vi "MacroEngine.vi"(11 "File Path":path=path "c:/RobotMacros.cfg") -> ()   [LabVIEW 2017]
uses:
  CtrlRefs/JoyStick1ALB.ctl
  CtrlRefs/JoyStick1ALV(Analog).ctl
  CtrlRefs/JoyStick2ALB.ctl
  CtrlRefs/JoyStick2ALB(Analog).ctl
  CtrlRefs/MacrosALB.ctl
  <vilib>/Rock Robotics/Network Tables/NT Write String Array.vi
  <vilib>/Rock Robotics/Network Tables/NT Write Boolean.vi
panel:
  out "MacroNames":string[](array[string])
  in  "DeleteMacroIndex":i32
  in  "DeleteMacro":bool
  in  "MacroRecStop":bool
  out "MacroRecording":bool
  out "MacroClock":dbl
  in  "MacroRecStart":bool
  in  "MacroName":string
  out "x*y":dbl
  out "Boolean":bool
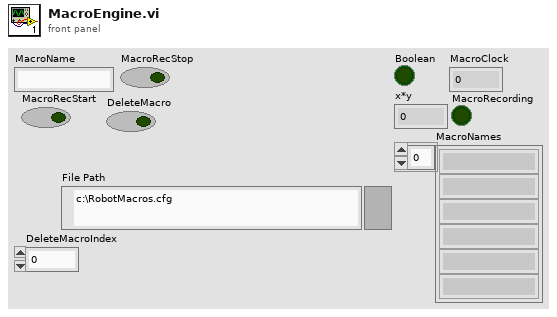
[diagram p1: front panel]
types:
  T1 = typedef "JoyStick1ALB.ctl" = cluster{"J1-B0":bool, "J1-B1":bool, "J1-B2":bool, "J1-B3":bool, "J1-B4":bool, "J1-B5":bool, "J1-B6":bool, "J1-B7":bool, "J1-B8-":bool, "J1-B9":bool, "J1-B10":bool, "J1-B11":bool}
  T2 = typedef "JoyStick1ALV(Analog).ctl" = cluster{"Axis 0":dbl, "Axis 1":dbl, "Axis 2":dbl, "Slider":dbl}
  T3 = typedef "JoyStick2ALB.ctl" = cluster{"J2-B0":bool, "J2-B1":bool, "J2-B2":bool, "J2-B3":bool, "J2-B4":bool, "J2-B5":bool, "J2-B6":bool, "J2-B7":bool, "J2-B8":bool, "J2-B9":bool, "J2-B10":bool, "J2-B11":bool}
  T4 = typedef "JoyStick2ALB(Analog).ctl" = cluster{"Axis 0":dbl, "Axis 1":dbl, "Axis 2":dbl, "Switch":dbl}
  T5 = cluster{"Buttons 1":T1, "Axes 1":T2, "Buttons 2":T3, "Axes 2":T4, "Delay":u32}
  T6 = cluster{"Buttons 1":T1, "Axes 1":T2, "Buttons 2":T3, "Axes 2":T4, "Delay":u32}[]
  T7 = typedef "MacrosALB.ctl" = cluster{"MacroName":string, "Sequence":cluster{"Buttons 1":T1, "Axes 1":T2, "Buttons 2":T3, "Axes 2":T4, "Delay":u32}[], "TotalTime":u32}
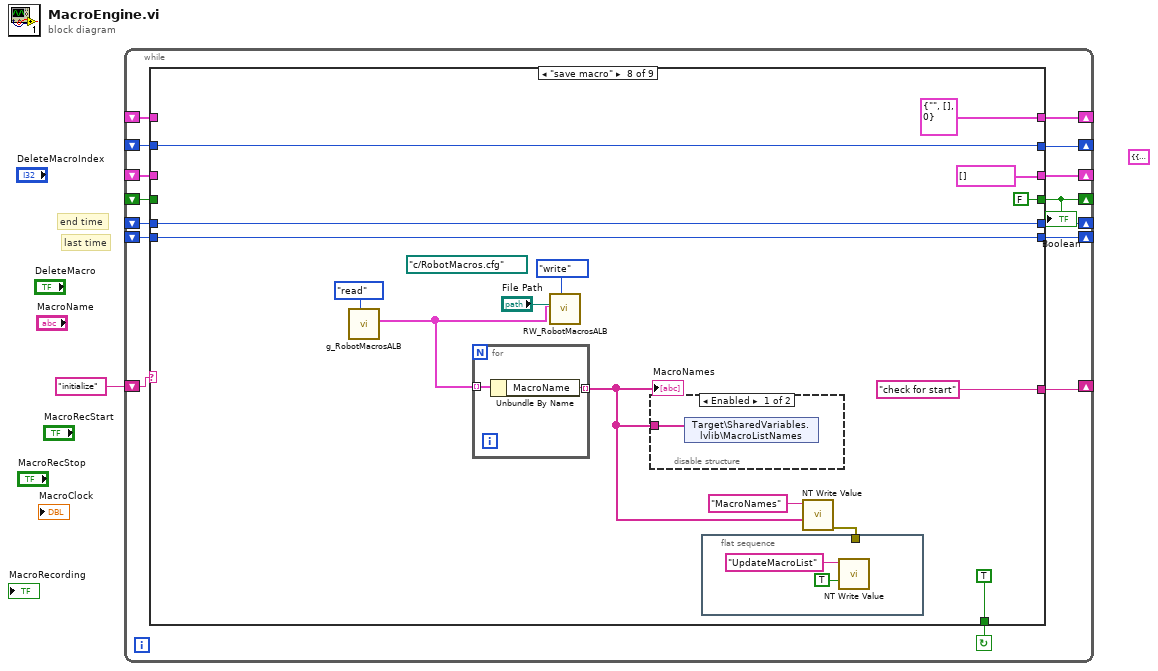
[diagram p0: block diagram]
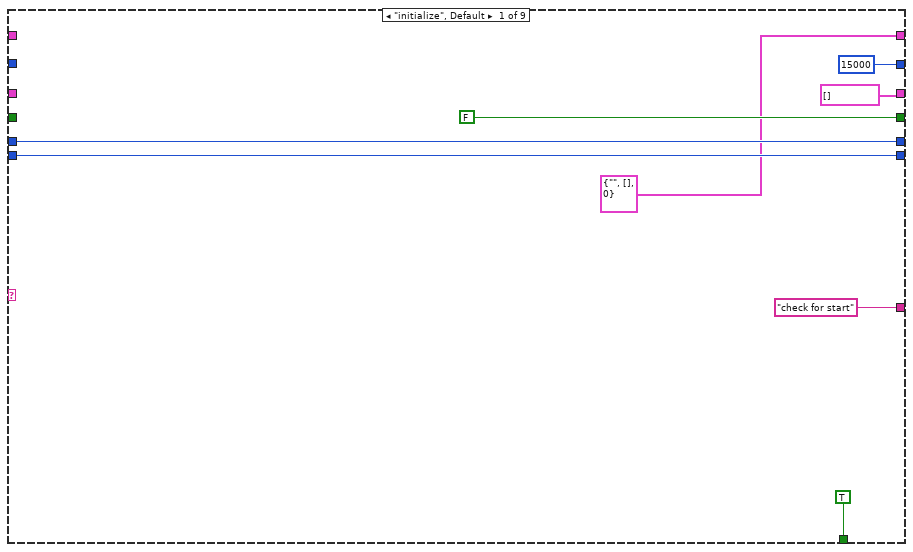
[diagram p2: hidden frame]
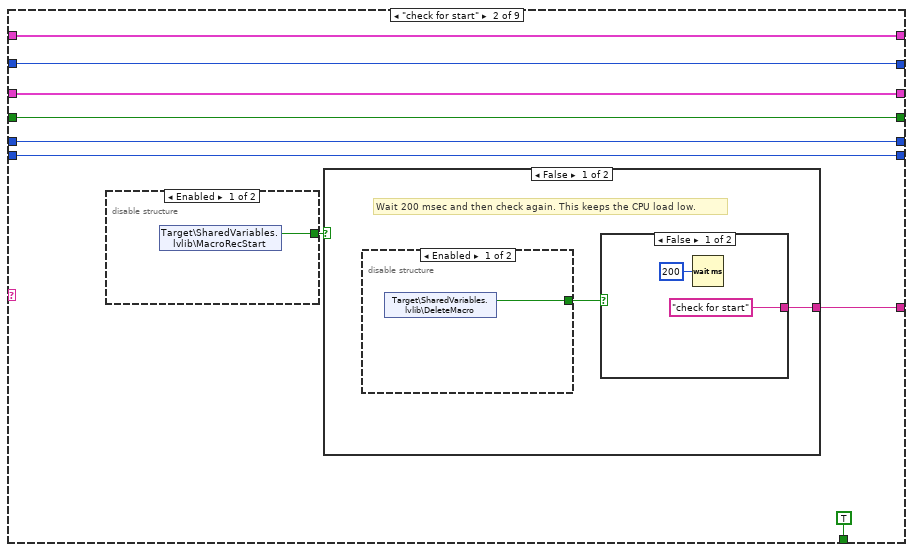
[diagram p3: hidden frame]
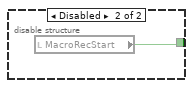
[diagram p4: hidden frame]
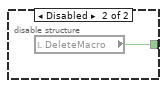
[diagram p5: hidden frame]
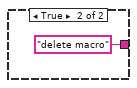
[diagram p6: hidden frame]
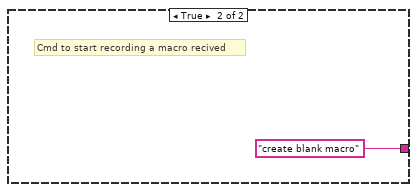
[diagram p7: hidden frame]
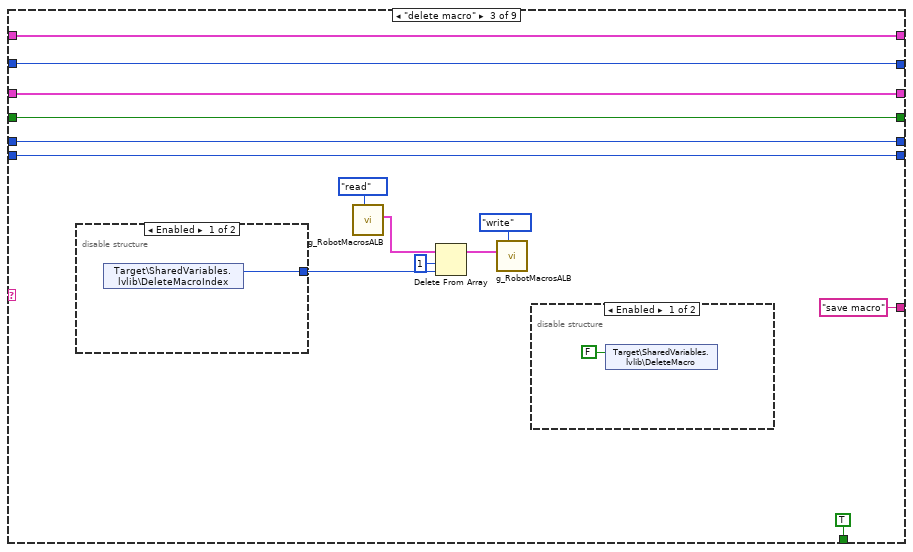
[diagram p8: hidden frame]
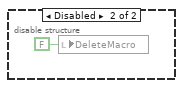
[diagram p9: hidden frame]
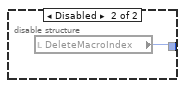
[diagram p10: hidden frame]
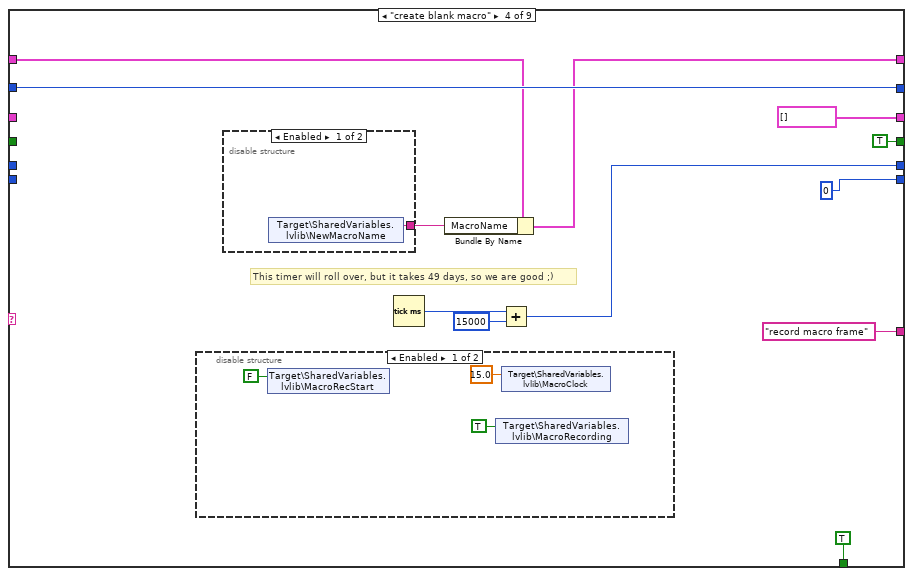
[diagram p11: hidden frame]
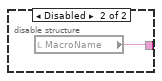
[diagram p12: hidden frame]
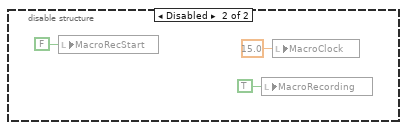
[diagram p13: hidden frame]
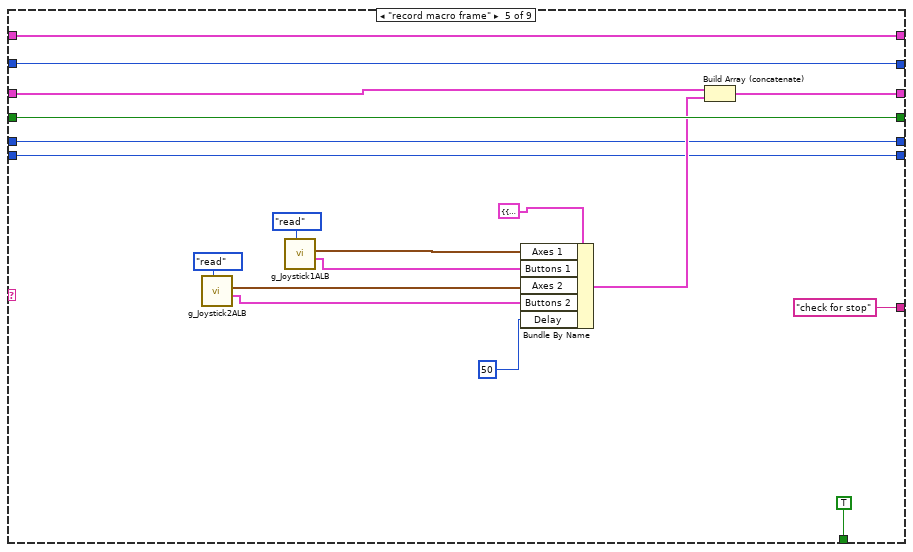
[diagram p14: hidden frame]
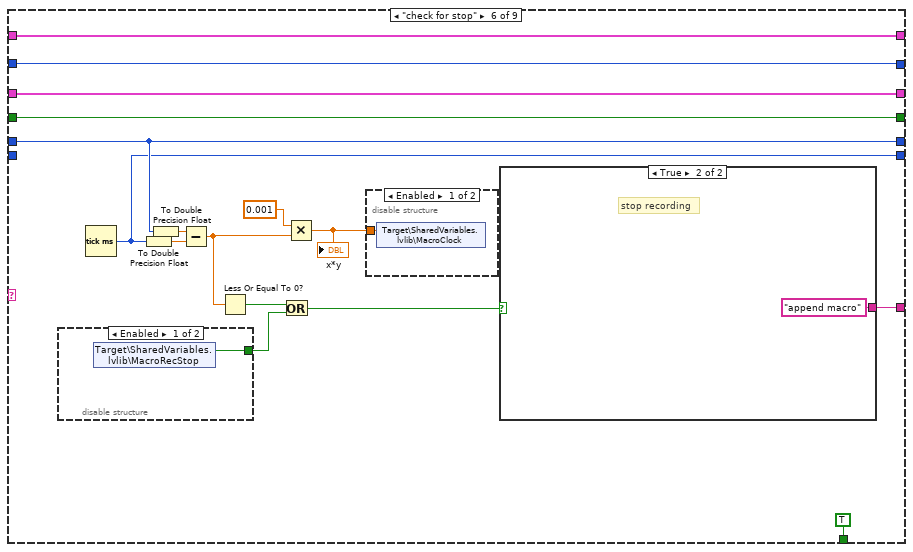
[diagram p15: hidden frame]
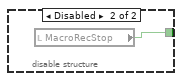
[diagram p16: hidden frame]
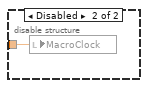
[diagram p17: hidden frame]
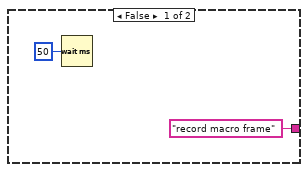
[diagram p18: hidden frame]
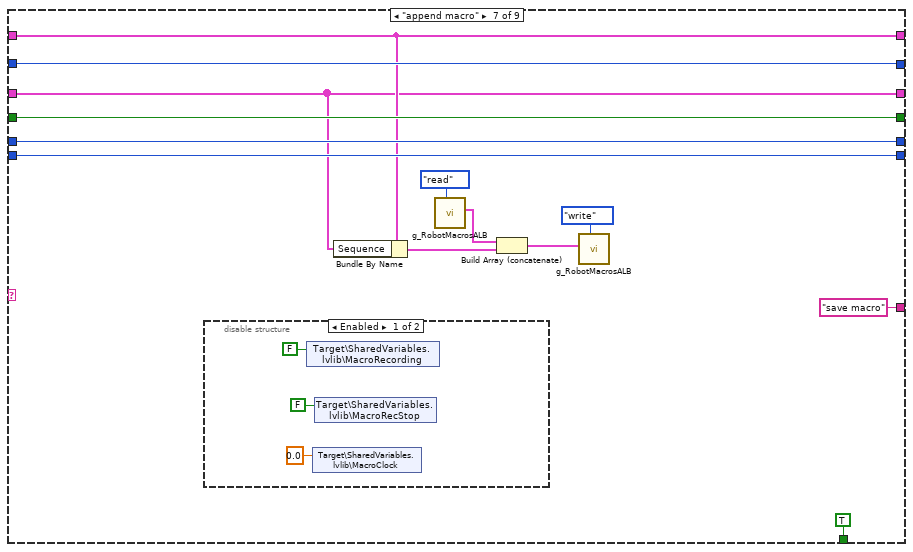
[diagram p19: hidden frame]
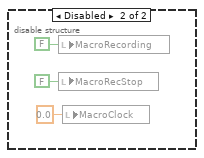
[diagram p20: hidden frame]
diagram:
  (unwired) T5 {"Buttons 1"={"J1-B0"=FALSE, "J1-B1"=FALSE, "J1-B2"=FALSE, "J1-B3"=FALSE, "J1-B4"=FALSE, "J1-B5"=FALSE, "J1-B6"=FALSE, "J1-B7"=FALSE, "J1-B8-"=FALSE, "J1-B9"=FALSE, "J1-B10"=FALSE, "J1-B11"=FALSE}, "Axes 1"={"Axis 0"=0.0, "Axis 1"=0.0, "Axis 2"=0.0, "Slider"=0.0}, "Buttons 2"={"J2-B0"=FALSE, "J2-B1"=FALSE, "J2-B2"=FALSE, "J2-B3"=FALSE, "J2-B4"=FALSE, "J2-B5"=FALSE, "J2-B6"=FALSE, "J2-B7"=FALSE, "J2-B8"=FALSE, "J2-B9"=FALSE, "J2-B10"=FALSE, "J2-B11"=FALSE}, "Axes 2"={"Axis 0"=0.0, "Axis 1"=0.0, "Axis 2"=0.0, "Switch"=0.0}, "Delay"=0} ("Segment")
  # "last time"
  # "end time"
  n1 = while {
    shift-right: [w12] -> _
    shift-left: "initialize" -> [w16]
    shift-right: [w15] -> _
    shift-left: _ -> [w14]
    shift-right: [w11] -> _
    shift-left: _ -> [w10]
    shift-right: [w9] -> _
    shift-left: _ -> [w8]
    shift-right: [w7] -> _
    shift-left: _ -> [w6]
    shift-right: [w5] -> _
    shift-left: _ -> [w4]
    shift-right: [w3] -> _
    shift-left: _ -> [w2]
    stop <- w13 continue-if-true
    n2 = case shown="\"save macro\"" w16 {
      tunnel: [15000 w33 w57 w73 w99 w115 w135 w156 w169] -> w15
      tunnel: w14 -> [_ w33 w57 w73 w99 w115 w135 w156 w169]
      tunnel: [TRUE TRUE TRUE TRUE TRUE TRUE TRUE TRUE FALSE] -> w13
      tunnel: ["check for start" w29 "save macro" "record macro frame" "check for stop" w103 "save macro" "check for start" "stop"] -> w12
      tunnel: [FALSE w32 w56 TRUE w98 w114 w134 FALSE w168] -> w11
      tunnel: w10 -> [_ w32 w56 _ w98 w114 w134 _ w168]
      tunnel: [T7 {"MacroName"="", "Sequence"=[], "TotalTime"=0} ("Macro") w28 w55 w68 w93 w113 w129 T7 {"MacroName"="", "Sequence"=[], "TotalTime"=0} ("Macro") w167] -> w9
      tunnel: w8 -> [_ w28 w55 w69 w93 w113 w129 _ w167]
      tunnel: [T6 [] ("Sequence") w27 w54 T6 [] ("Sequence") w91 w104 w128 T6 [] ("Sequence") w166] -> w7
      tunnel: w6 -> [_ w27 w54 _ w92 w104 w128 _ w166]
      tunnel: [w20 w26 w53 w67 w84 w106 w133 w151 w165] -> w5
      tunnel: w4 -> [w20 w26 w53 _ w84 w106 w133 w151 w165]
      tunnel: [w19 w25 w52 u32 0 ("millisecond timer value") w83 w102 w132 w150 w164] -> w3
      tunnel: w2 -> [w19 w25 w52 _ w83 _ w132 w150 w164]
      frame "initialize", Default {
      }
      frame "check for start" {
        n3 = disable-structure shown="Enabled" {
          disable-tunnel: [w34 w35] -> w30
          frame Enabled {
            n4 = shared-variable "Target\\SharedVariables.lvlib\\MacroRecStart"() -> (w34:bool)  [unwired: 1 in, 1 out]
          }
          frame Disabled {
            n5 = local read "MacroRecStart"() -> (w35:bool)
          }
        }
        n6 = case shown="False" w30 {
          tunnel: [w37 "create blank macro"] -> w29
          frame False {
            # "Wait 200 msec and then check again. This keeps the CPU load low."
            n7 = disable-structure shown="Enabled" {
              disable-tunnel: [w38 w39] -> w36
              frame Enabled {
                n8 = shared-variable "Target\\SharedVariables.lvlib\\DeleteMacro"() -> (w38:bool)  [unwired: 1 in, 1 out]
              }
              frame Disabled {
                n9 = local read "DeleteMacro"() -> (w39:bool)
              }
            }
            n10 = case shown="False" w36 {
              tunnel: ["check for start" "delete macro"] -> w37
              frame False {
                n11 = Wait (ms)(milliseconds to wait=u32 200) -> ()  [unwired: 1 out]
              }
              frame True {
              }
            }
          }
          frame True {
            # "Cmd to start recording a macro recived"
          }
        }
      }
      frame "delete macro" {
        n12 = disable-structure shown="Enabled" {
          disable-tunnel: [w60 w61] -> w45
          frame Enabled {
            n13 = shared-variable "Target\\SharedVariables.lvlib\\DeleteMacroIndex"() -> (w60:i32)  [unwired: 1 in, 1 out]
          }
          frame Disabled {
            n14 = local read "DeleteMacroIndex"() -> (w61:i32)
          }
        }
        n15 = call "g_RobotMacrosALB.vi"("Action"=enum16{"read", "write"}."read") -> ("Macros out"=w47:T7[])  [unwired: 10 in]
        n16 = Delete From Array(array=w47, length=1, index=w45) -> (array with subset deleted=w44:T7[])  [unwired: 1 out]
        n17 = call "g_RobotMacrosALB.vi"("Action"=enum16{"read", "write"}."write", "Macros"=w44) -> ()  [unwired: 9 in, 1 out]
        n18 = disable-structure shown="Enabled" {
          frame Enabled {
            n19 = shared-variable "Target\\SharedVariables.lvlib\\DeleteMacro"(FALSE ("DeleteMacro")) -> ()  [unwired: 1 in, 1 out]
          }
          frame Disabled {
            n20 = local write "DeleteMacro"(FALSE ("DeleteMacro")) -> ()
          }
        }
      }
      frame "create blank macro" {
        # "This timer will roll over, but it takes 49 days, so we are good ;)"
        n21 = disable-structure shown="Enabled" {
          frame Enabled {
            n22 = shared-variable "Target\\SharedVariables.lvlib\\MacroRecStart"(FALSE ("MacroRecStart")) -> ()  [unwired: 1 in, 1 out]
            n23 = shared-variable "Target\\SharedVariables.lvlib\\MacroRecording"(TRUE ("MacroRecording")) -> ()  [unwired: 1 in, 1 out]
            n24 = shared-variable "Target\\SharedVariables.lvlib\\MacroClock"(15.0 ("MacroClock")) -> ()  [unwired: 1 in, 1 out]
          }
          frame Disabled {
            n25 = local write "MacroRecStart"(FALSE ("MacroRecStart")) -> ()
            n26 = local write "MacroRecording"(TRUE ("MacroRecording")) -> ()
            n27 = local write "MacroClock"(15.0 ("MacroClock")) -> ()
          }
        }
        n28 = disable-structure shown="Enabled" {
          disable-tunnel: [w74 w75] -> w70
          frame Enabled {
            n29 = shared-variable "Target\\SharedVariables.lvlib\\NewMacroName"() -> (w74:string)  [unwired: 1 in, 1 out]
          }
          frame Disabled {
            n30 = local read "MacroName"() -> (w75:string)
          }
        }
        n31 = Tick Count (ms)() -> (millisecond timer value=w65:u32)
        n32 = Bundle By Name(cluster=w69, "MacroName"=w70) -> (w68:T7)
        n33 = Add(x=w65, y=u32 15000) -> (x+y=w67:u32)
      }
      frame "record macro frame" {
        n34 = call "g_Joystick2ALB.vi"("Action"=enum16{"initialize", "read", "write"}."read") -> ("Buttons out"=w86:T3, "Axes out"=w87:T4)  [unwired: 7 in, 2 out]
        n35 = call "g_Joystick1ALB.vi"("Action"=enum16{"initialize", "read", "write"}."read") -> ("Buttons out"=w89:T1, "Axes out"=w90:T2)  [unwired: 7 in, 2 out]
        n36 = Bundle By Name(cluster=T5 {"Buttons 1"={"J1-B0"=FALSE, "J1-B1"=FALSE, "J1-B2"=FALSE, "J1-B3"=FALSE, "J1-B4"=FALSE, "J1-B5"=FALSE, "J1-B6"=FALSE, "J1-B7"=FALSE, "J1-B8-"=FALSE, "J1-B9"=FALSE, "J1-B10"=FALSE, "J1-B11"=FALSE}, "Axes 1"={"Axis 0"=0.0, "Axis 1"=0.0, "Axis 2"=0.0, "Slider"=0.0}, "Buttons 2"={"J2-B0"=FALSE, "J2-B1"=FALSE, "J2-B2"=FALSE, "J2-B3"=FALSE, "J2-B4"=FALSE, "J2-B5"=FALSE, "J2-B6"=FALSE, "J2-B7"=FALSE, "J2-B8"=FALSE, "J2-B9"=FALSE, "J2-B10"=FALSE, "J2-B11"=FALSE}, "Axes 2"={"Axis 0"=0.0, "Axis 1"=0.0, "Axis 2"=0.0, "Switch"=0.0}, "Delay"=0} ("Segment"), "Axes 1"=w90, "Buttons 1"=w89, "Axes 2"=w87, "Buttons 2"=w86, "Delay"=u32 50) -> (w94:T5)
        n37 = Build Array (concatenate)(w92, w94) -> (w91:T6)
      }
      frame "check for stop" {
        n38 = disable-structure shown="Enabled" {
          disable-tunnel: [w116 w117] -> w109
          frame Enabled {
            n39 = shared-variable "Target\\SharedVariables.lvlib\\MacroRecStop"() -> (w116:bool)  [unwired: 1 in, 1 out]
          }
          frame Disabled {
            n40 = local read "MacroRecStop"() -> (w117:bool)
          }
        }
        n41 = Tick Count (ms)() -> (millisecond timer value=w102:u32)
        n42 = To Double Precision Float(number=w102) -> (double precision float=w100:dbl)
        n43 = To Double Precision Float(number=w106) -> (double precision float=w101:dbl)
        n44 = Subtract(x=w101, y=w100) -> (x-y=w108:dbl)
        n45 = Less Or Equal To 0?(x=w108) -> (x <= 0?=w110:bool)
        n46 = Or(x=w110, y=w109) -> (x .or. y?=w105:bool)
        n47 = Multiply(x=0.001, y=w108) -> (x*y=w107:dbl)
        "x*y" <- w107
        n48 = disable-structure shown="Enabled" {
          disable-tunnel: w107 -> [w118 w119]
          frame Enabled {
            n49 = shared-variable "Target\\SharedVariables.lvlib\\MacroClock"(w118) -> ()  [unwired: 1 in, 1 out]
          }
          frame Disabled {
            n50 = local write "MacroClock"(w119) -> ()
          }
        }
        n51 = case shown="True" w105 {
          tunnel: ["record macro frame" "append macro"] -> w103
          frame False {
            n52 = Wait (ms)(milliseconds to wait=u32 50) -> ()  [unwired: 1 out]
          }
          frame True {
            # "stop recording"
          }
        }
      }
      frame "append macro" {
        n53 = disable-structure shown="Enabled" {
          frame Enabled {
            n54 = shared-variable "Target\\SharedVariables.lvlib\\MacroRecording"(FALSE ("MacroRecording")) -> ()  [unwired: 1 in, 1 out]
            n55 = shared-variable "Target\\SharedVariables.lvlib\\MacroClock"(0.0 ("MacroClock")) -> ()  [unwired: 1 in, 1 out]
            n56 = shared-variable "Target\\SharedVariables.lvlib\\MacroRecStop"(FALSE ("MacroRecStop")) -> ()  [unwired: 1 in, 1 out]
          }
          frame Disabled {
            n57 = local write "MacroRecording"(FALSE ("MacroRecording")) -> ()
            n58 = local write "MacroRecStop"(FALSE ("MacroRecStop")) -> ()
            n59 = local write "MacroClock"(0.0 ("MacroClock")) -> ()
          }
        }
        n60 = Bundle By Name(cluster=w129, "Sequence"=w128) -> (w127:T7)
        n61 = call "g_RobotMacrosALB.vi"("Action"=enum16{"read", "write"}."read") -> ("Macros out"=w124:T7[])  [unwired: 10 in]
        n62 = Build Array (concatenate)(w124, w127) -> (w123:T7[])
        n63 = call "g_RobotMacrosALB.vi"("Action"=enum16{"read", "write"}."write", "Macros"=w123) -> ()  [unwired: 9 in, 1 out]
      }
      frame "save macro" {
        (unwired) path "c:/RobotMacros.cfg" ("File Path")
        n64 = call "g_RobotMacrosALB.vi"("Action"=enum16{"read", "write"}."read") -> ("Macros out"=w145:T7[])  [unwired: 10 in]
        n65 = for {
          tunnel: w145 -> [w161] mode=indexing
          tunnel: [w160] -> w142 mode=indexing
          n66 = Unbundle By Name(w161) -> ("MacroName"=w160:string)
        }
        "MacroNames" <- w142
        n67 = call "RW_RobotMacrosALB.vi"("Action"=enum16{"read", "write"}."write", "Macros"=w145, "File Path"="File Path") -> ()  [unwired: 7 in, 2 out]
        n68 = disable-structure shown="Enabled" {
          disable-tunnel: w142 -> [w157 _]
          frame Enabled {
            n69 = shared-variable "Target\\SharedVariables.lvlib\\MacroListNames"(w157) -> ()  [unwired: 1 in, 1 out]
          }
          frame Disabled {
          }
        }
        n70 = flat-sequence {
          tunnel: w143 -> [_]
          frame #0 {
            n71 = call-poly <vilib>:"NT Write Value.vi"("Boolean"=TRUE ("Default Value"), "Name"="UpdateMacroList") -> ()  [unwired: 9 in, 1 out]
          }
        }
        n72 = call-poly <vilib>:"NT Write Value.vi"("String Array"=w142, "Name"="MacroNames") -> ("error out"=w143:errorcluster)  [unwired: 9 in]
      }
      frame "stop" {
      }
    }
    "Boolean" <- w11
  }
